vi "getImageTempsamples.vi"(8 "error in (no error)":errorcluster, 11 "params":refnum<class "JSON Value.lvclass">) -> (0 "error out":errorcluster, 3 "data":refnum<class "JSON Value.lvclass">)   [LabVIEW 2017]
uses:
  <vilib>/NI/JSON Support for LabVIEW/JSON Value/JSON Value.lvclass
  ax5.lvclass
  <vilib>/NI/JSON Support for LabVIEW/JSON Value/Object/Get Value/Get Value (String).vi
  <vilib>/NI/JSON Support for LabVIEW/JSON Value/Object/Get Value/Get Value (Numeric).vi
  <vilib>/NI/JSON Support for LabVIEW/JSON Value/New JSON Value/New JSON (Numeric[]).vi
  <vilib>/NI/JSON Support for LabVIEW/JSON Value/New JSON Value/New JSON ({Value[]}).vi
  <vilib>/NI/NI JSONRPC Server Framework/Classes/Server/JSONRPC Server.lvclass
panel:
  out "Image Data":dbl[][](array[numeric])
  in  "emissivity":dbl=0.6
  in  "camera":string="cam0"
  in  "Debug":bool
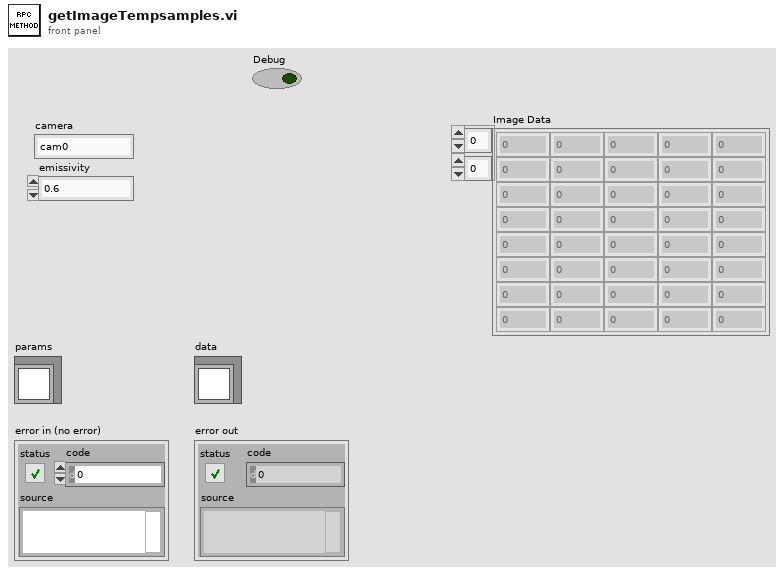
[diagram p1: front panel]
types:
  T1 = typedef "Image Type" = u32
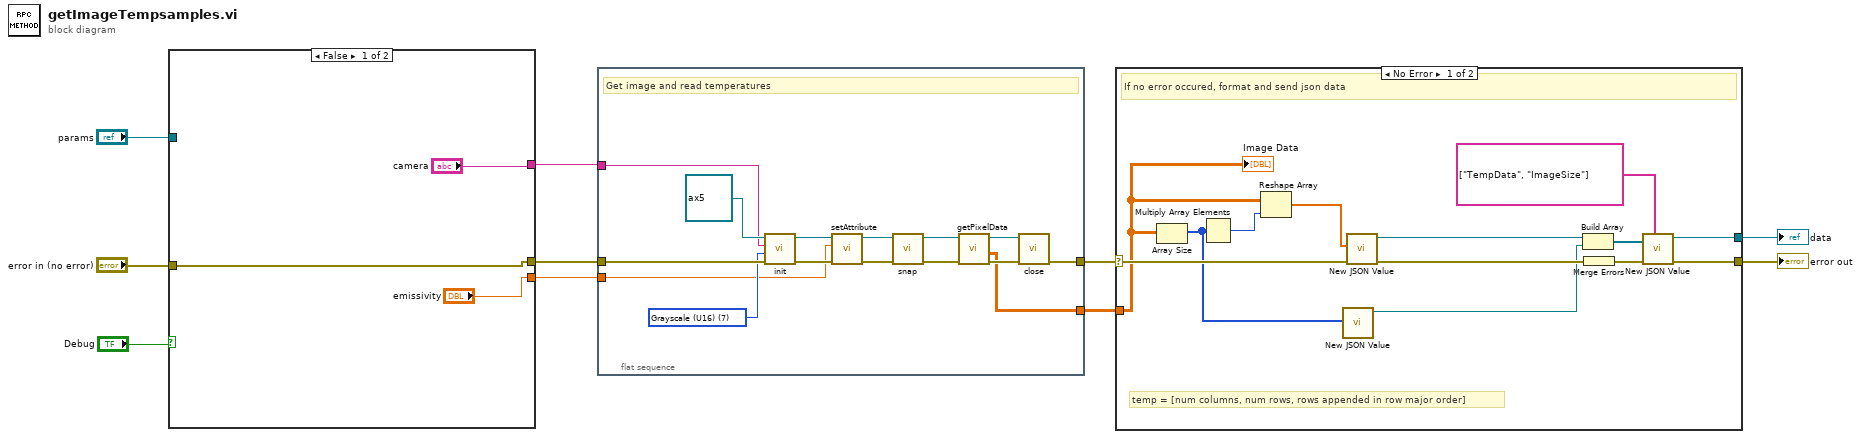
[diagram p0: block diagram]
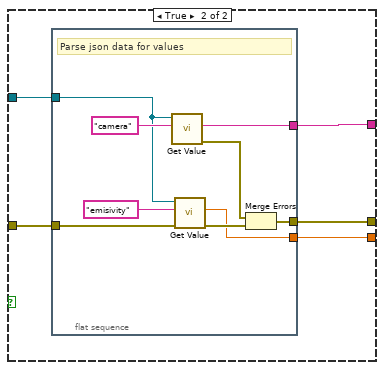
[diagram p2: hidden frame]
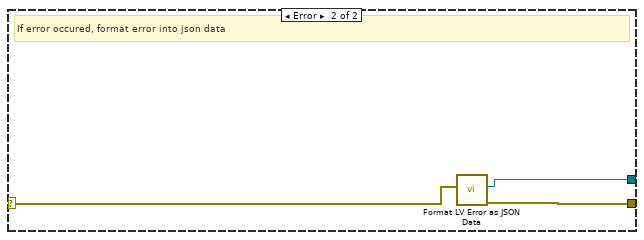
[diagram p3: hidden frame]
diagram:
  n1 = case shown="False" "Debug" {
    tunnel: "params" -> [_ w18]
    tunnel: "error in (no error)" -> [w12 w17]
    tunnel: [w12 w16] -> w4
    tunnel: ["camera" w15] -> w3
    tunnel: ["emissivity" w14] -> w2
    frame False {
    }
    frame True {
      n2 = flat-sequence {
        tunnel: w18 -> [w25]
        tunnel: w17 -> [w24]
        tunnel: [w21] -> w16
        tunnel: [w20] -> w15
        tunnel: [w19] -> w14
        frame #0 {
          # "Parse json data for values"
          n3 = call-poly <vilib>:"Get Value.vi"("key"="camera", "JSON Value in"=w25) -> ("error out"=w22:errorcluster, "value"=w20:string)  [unwired: 8 in]
          n4 = call-poly <vilib>:"Get Value.vi"("error in (no error)"=w24, "key"="emisivity", "JSON Value in"=w25) -> ("error out"=w23:errorcluster, "value"=w19:dbl)  [unwired: 7 in]
          n5 = Merge Errors(w22, w23) -> (w21:errorcluster)
        }
      }
    }
  }
  n6 = flat-sequence {
    tunnel: w4 -> [w42]
    tunnel: w3 -> [w40]
    tunnel: [w30] -> w8
    tunnel: [w29] -> w5
    tunnel: w2 -> [w28]
    frame #0 {
      w39 = T1 7 items=["Grayscale (U8)", "Grayscale (I16)", "Grayscale (SGL)", "Complex (CSG)", "RGB (U32)", "HSL (U32)", "RGB (U64)", "Grayscale (U16)"] ("Image Type")
      # "Get image and read temperatures"
      n7 = call-dynamic "init.vi"("error in (no error)"=w42, "Image Type"=w39, "Camera Name"=w40, "ax5 in"=refnum<class "ax5.lvclass"> refnum ("ax5.lvclass")) -> ("error out"=w38:errorcluster, "ax5 out"=w37:refnum<class "ax5.lvclass">)  [unwired: 6 in]
      n8 = call-dynamic "setAttribute.vi"("error in (no error)"=w38, "Emissivity"=w28, "ax5.lvclass"=w37) -> ("error out"=w35:errorcluster, "ax5.lvclass"=w36:refnum<class "ax5.lvclass">)  [unwired: 7 in]
      n9 = call-dynamic "snap.vi"("error in (no error)"=w35, "camera in"=w36) -> ("error out"=w34:errorcluster, "camera out"=w33:refnum<class "ax5.lvclass">)  [unwired: 7 in, 1 out]
      n10 = call-dynamic "getPixelData.vi"("error in (no error)"=w34, "ax5 in"=w33) -> ("error out"=w32:errorcluster, "Temp"=w29:dbl[][], "ax5 out"=w31:refnum<class "ax5.lvclass">)  [unwired: 5 in, 2 out]
      n11 = call-dynamic "close.vi"("error in (no error)"=w32, "camera in"=w31) -> ("error out"=w30:errorcluster)  [unwired: 8 in, 1 out]
    }
  }
  n12 = case shown="No Error" w8 {
    selector: w8 -> [w51 w58]
    tunnel: [w54 w56] -> w7
    tunnel: [w50 w57] -> w6
    tunnel: w5 -> [w43 _]
    frame No Error {
      # "temp = [num columns, num rows, rows appended in row major order]"
      # "If no error occured, format and send json data"
      n13 = Array Size(array=w43) -> (size(s)=w44:i32[])
      n14 = Multiply Array Elements(1:w44) -> (0:w46:i32)
      n15 = Reshape Array(w43, w46) -> (w45:dbl[])
      n16 = call-poly <vilib>:"New JSON Value.vi"("Numeric Array"=w44) -> ("JSON Value out"=w47:refnum<class "JSON Value.lvclass">)  [unwired: 9 in, 1 out]
      n17 = call-poly <vilib>:"New JSON Value.vi"("error in (no error)"=w51, "Numeric Array"=w45) -> ("error out"=w55:errorcluster, "JSON Value out"=w53:refnum<class "JSON Value.lvclass">)  [unwired: 8 in]
      n18 = Build Array(w53, w47) -> (w49:refnum<class "JSON Value.lvclass">[])
      n19 = Merge Errors(w55) -> (w52:errorcluster)
      n20 = call-poly <vilib>:"New JSON Value.vi"("keys"=string[] ["TempData", "ImageSize"], "error in (no error)"=w52, "values"=w49) -> ("error out"=w54:errorcluster, "JSON Value out"=w50:refnum<class "JSON Value.lvclass">)  [unwired: 7 in]
      "Image Data" <- w43
    }
    frame Error {
      # "If error occured, format error into json data"
      n21 = call <vilib>:"Format LV Error as JSON Data.vi"("error in"=w58) -> ("error out"=w56:errorcluster, "Error Value out"=w57:refnum<class "JSON Value.lvclass">)  [unwired: 9 in]
    }
  }
  "data" <- w6
  "error out" <- w7
